vi "PV Software Temperature Conversion.vi"(10 "HEX Data (Byte 2)":u8 format="%.0x", 11 "HEX Data (Byte 1)":u8 format="%.0x") -> (3 "Temperature (F)":string)   [LabVIEW 2023]
panel:
  out "x+y":u16
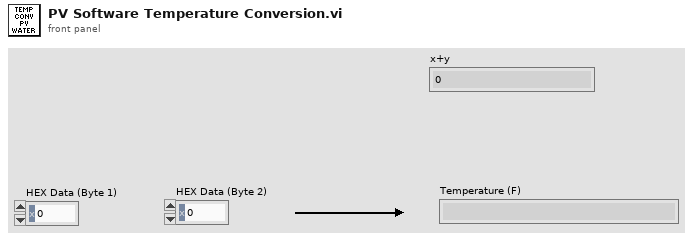
[diagram p1: front panel]
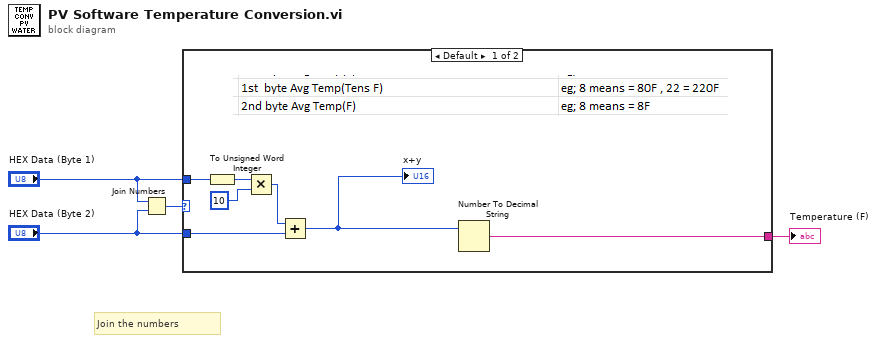
[diagram p0: block diagram]
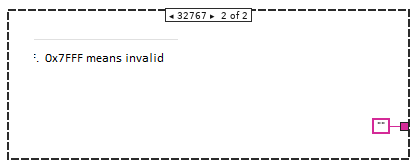
[diagram p2: hidden frame]
diagram:
  # "Join the numbers"
  n1 = Join Numbers(hi="HEX Data (Byte 1)", lo="HEX Data (Byte 2)") -> ((hi.lo)=w4:u16)
  n2 = case shown="Default" w4 {
    tunnel: [w8 ""] -> w1
    tunnel: "HEX Data (Byte 2)" -> [w7 _]
    tunnel: "HEX Data (Byte 1)" -> [w6 _]
    frame Default {
      n3 = To Unsigned Word Integer(number=w6) -> (unsigned 16bit integer=w5:u16)
      n4 = Multiply(x=w5, y=u16 10) -> (x*y=w10:u16)
      n5 = Add(x=w10, y=w7) -> (x+y=w11:u16)
      "x+y" <- w11
      n6 = Number To Decimal String(number=w11) -> (decimal integer string=w8:string)  [unwired: 1 in]
    }
    frame 32767 {
    }
  }
  "Temperature (F)" <- w1
